vi "SW_Fire_TTL_at_stop_universal.vi"(6 "TTL port(s) config to fire":u8, 7 "TTL pulse length, ms":dbl=250.0 format="%#_13g", 8 "error in (no error)":errorcluster, 9 "Serial Port In":refnum<visa-resource-name>="COM3", 10 "Close VISA (T)":bool=TRUE, 11 "Start/stop signaling (F)":bool) -> (0 "error out":errorcluster, 1 "Serial Port Out":refnum<visa-resource-name>="COM3", 3 "Time spent to process command, ms":dbl=250.0)   [LabVIEW 2016]
doc: "Fires TTL High to the TTL2 output for ~250 ms (default)."
uses:
  <vilib>/Instr/_visa.llb/VISA Flush IO Buffer Mask.ctl
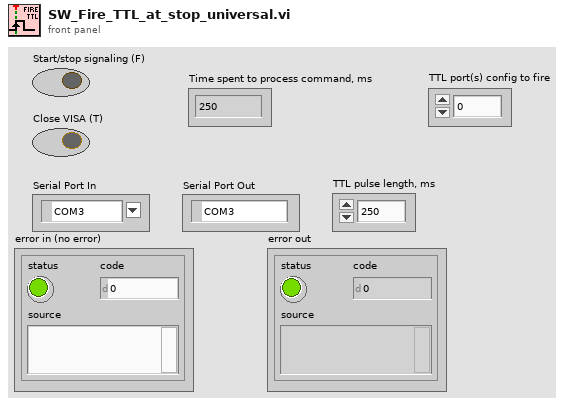
[diagram p1: front panel]
types:
  T1 = typedef "VISA Flush IO Buffer Mask.ctl" = u16
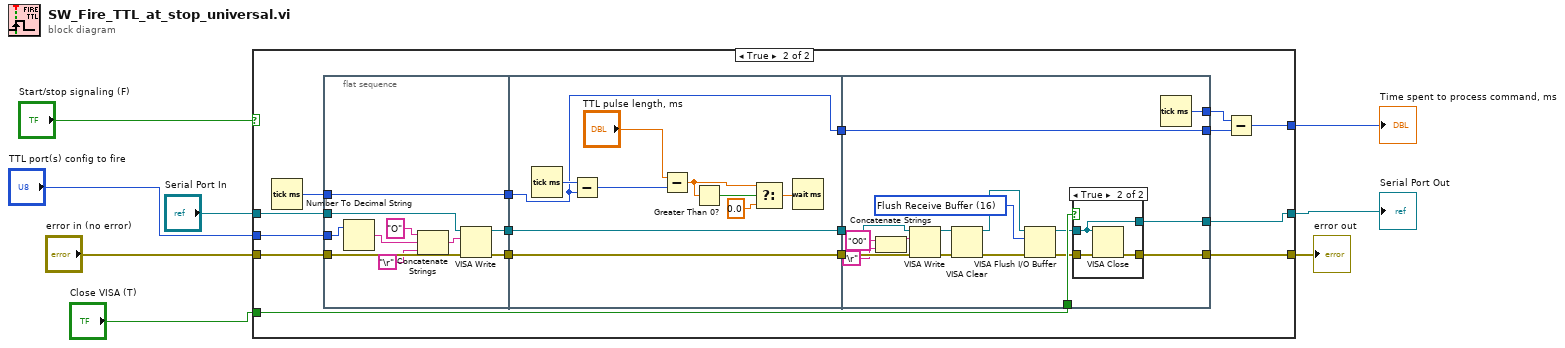
[diagram p0: block diagram]
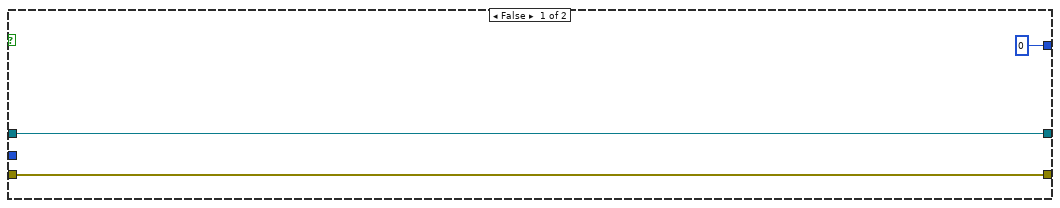
[diagram p2: hidden frame]
diagram:
  n1 = case shown="True" "Start/stop signaling (F)" {
    tunnel: [u32 0 w18] -> w8
    tunnel: [w10 w17] -> w7
    tunnel: "Serial Port In" -> [w10 w16]
    tunnel: "Close VISA (T)" -> [_ w15]
    tunnel: [w9 w14] -> w3
    tunnel: "error in (no error)" -> [w9 w13]
    tunnel: "TTL port(s) config to fire" -> [_ w12]
    frame False {
    }
    frame True {
      n2 = Tick Count (ms)() -> (millisecond timer value=w22:u32)
      n3 = flat-sequence {
        tunnel: w16 -> [w35]
        tunnel: [w37] -> w27
        tunnel: [w36] -> w26
        tunnel: [w34] -> w23
        tunnel: w22 -> [w34]
        tunnel: w13 -> [w33]
        tunnel: w12 -> [w30]
        tunnel: [w47] -> w25
        tunnel: w27 -> [w47]
        tunnel: [w46] -> w24
        tunnel: w26 -> [w46]
        tunnel: w23 -> [w38]
        tunnel: [w38] -> w19
        tunnel: [w61] -> w14
        tunnel: [w62] -> w17
        tunnel: [w63] -> w20
        tunnel: [w64] -> w21
        tunnel: w15 -> [w60]
        tunnel: w19 -> [w63]
        tunnel: w24 -> [w54]
        tunnel: w25 -> [w53]
        frame #0 {
          n4 = Number To Decimal String(number=w30) -> (decimal integer string=w32:string)  [unwired: 1 in]
          n5 = Concatenate Strings("O" ("string"), w32, "\r") -> (w29:string)
          n6 = VISA Write(VISA resource name=w35, write buffer=w29, error in (no error)=w33) -> (VISA resource name out=w37:refnum<visa-resource-name>, error out=w36:errorcluster)  [unwired: 1 out]
        }
        frame #1 {
          n7 = Tick Count (ms)() -> (millisecond timer value=w45:u32)
          n8 = Subtract(x=w45, y=w38) -> (x-y=w43:u32)
          n9 = Subtract(x="TTL pulse length, ms", y=w43) -> (x-y=w40:dbl)
          n10 = Greater Than 0?(x=w40) -> (x > 0?=w42:bool)
          n11 = Select(t=w40, s=w42, f=0.0) -> (s? t:f=w41:dbl)
          n12 = Wait (ms)(milliseconds to wait=w41) -> ()  [unwired: 1 out]
        }
        frame #2 {
          w55 = T1 16 items=["Flush Receive Buffer"=16, "Write Transmit Buffer to Device"=32, "Flush Receive Buffer (No I/O)"=64, "Flush Transmit Buffer"=128] ("Mask")
          n13 = Concatenate Strings("O0" ("string"), "\r") -> (w49:string)
          n14 = VISA Write(VISA resource name=w53, write buffer=w49, error in (no error)=w54) -> (VISA resource name out=w52:refnum<visa-resource-name>, error out=w51:errorcluster)  [unwired: 1 out]
          n15 = VISA Clear(VISA resource name=w52, error in (no error)=w51) -> (VISA resource name out=w57:refnum<visa-resource-name>, error out=w59:errorcluster)
          n16 = VISA Flush I/O Buffer(VISA resource name=w57, mask (16)=w55, error in (no error)=w59) -> (VISA resource name out=w56:refnum<visa-resource-name>, error out=w58:errorcluster)
          n17 = case shown="True" w60 {
            tunnel: w56 -> [w66 w68]
            tunnel: w58 -> [w65 w67]
            tunnel: [w66 w68] -> w62
            tunnel: [w65 w69] -> w61
            frame False {
            }
            frame True {
              n18 = VISA Close(VISA resource name=w68, error in (no error)=w67) -> (error out=w69:errorcluster)
            }
          }
          n19 = Tick Count (ms)() -> (millisecond timer value=w64:u32)
        }
      }
      n20 = Subtract(x=w21, y=w20) -> (x-y=w18:u32)
    }
  }
  "Time spent to process command, ms" <- w8
  "Serial Port Out" <- w7
  "error out" <- w3
